vi "Rotation_Times.vi"(9 "Scalar":dbl, 11 "in ROTATION":T1) -> (3 "out ROTATION":T1)   [LabVIEW 2019, in "Trajectory_Library.lvlib"]
doc: "Multiplies the current rotation (angle) by a scalar.\n\nParameters: \n- IN ROTATION - This ROTATION data structure\n- SCALAR - The value to multiiply the rotation by.\n\nReturns:\n - OUT ROTATION - THe new ROTATION data structure."
uses:
  Trajectory_Library.lvlib
  ROTATION2D.ctl
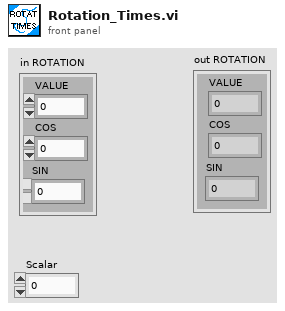
[diagram p1: front panel]
types:
  T1 = typedef "Trajectory_Library.lvlib/ROTATION2D.ctl" = cluster{"VALUE":dbl, "COS":dbl, "SIN":dbl}
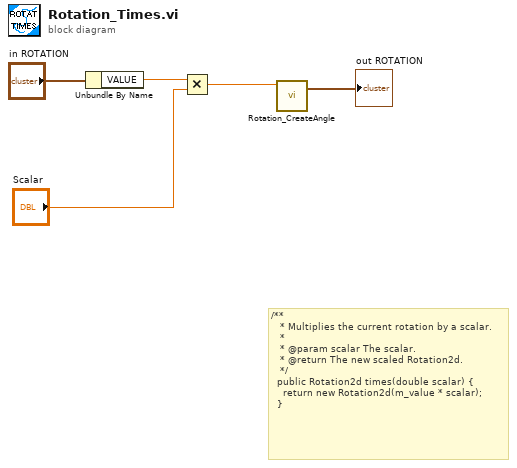
[diagram p0: block diagram]
diagram:
  # "/**\n   * Multiplies the current rotation by a scalar.\n   *\n   * @param scalar The scalar.\n   * @return The new scaled Rotation2d.\n   */\n  public Rotation2d times(double scalar) {\n    return new Rotation2d(m_value * scalar);\n  }"
  n1 = Unbundle By Name("in ROTATION") -> ("VALUE"=w4:dbl)
  n2 = Multiply(x=w4, y="Scalar") -> (x*y=w2:dbl)
  n3 = call "Rotation_CreateAngle.vi"("Angle"=w2) -> ("ROTATION"=→"out ROTATION":T1)  [unwired: 10 in]
